vi "Main (429).vi"() -> ()   [LabVIEW 2020]
doc: "Use this template to build a simple state machine design pattern. Each state executes code and determines which state to transition to."
uses:
  Controls/State.ctl
  Controls/Data.ctl
  Controls/Database_Array.ctl
  Controls/Encoding.ctl
  <vilib>/Utility/error.llb/DialogType.ctl
  <userlib>/_OpenG.lib/array/array.llb/Remove Duplicates from 1D Array (I32)__ogtk.vi
  <userlib>/_OpenG.lib/array/array.llb/Sort 1D Array (I32)__ogtk.vi
  <userlib>/_OpenG.lib/array/array.llb/Search 1D Array (I32)__ogtk.vi
  <userlib>/_OpenG.lib/array/array.llb/Index 1D Array Elements (Variant)__ogtk.vi
  Libraries/Ballard_429_Parameter_ni/Ballard_429_Parameter_ni.lvlib
  Libraries/Aim_429_Parameter_ni/AIM_429_Parameter_ni.lvlib
panel:
  in  "formatting":enum16{"NIVeriStandAdd-Ons", "ni", "ni-AIM"}(ring)
  in  "Configure SelfTestBus?":bool
  out "Progress":string
  in  "Stop Button":bool
  in  "Generate XMLs":bool
  in  "Database Filepath (xlsx)":path
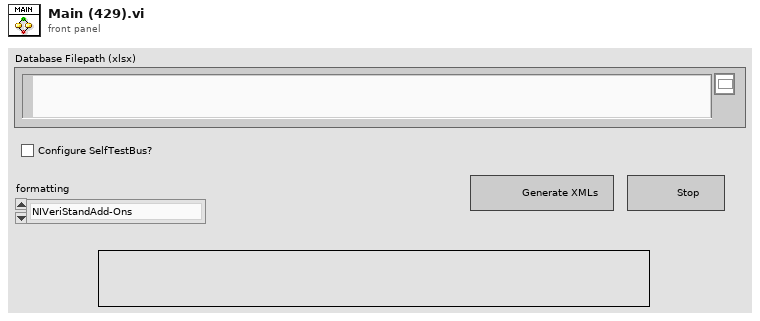
[diagram p1: front panel]
types:
  T1 = typedef "DialogType.ctl" = u16
  T2 = typedef "Data.ctl" = cluster{"Cores to Process Array":i32[], "All Parameters Array":T3[], "Filtered Parameter Array":T3[], "Core Number":i32, "Database Filepath (xlsx)":path, "Selected Self Test Channels":i32[], "formatting":enum16{"NIVeriStandAdd-Ons", "ni", "ni-AIM"}}
  T3 = typedef "Database_Array.ctl" = cluster{"Core Number":i32, "Channel Number":i32, "Channel Name":string, "Channel Speed":i32, "Label Decimal":i32, "Label Name":string, "Min Rate (mS)":i32, "Max Rate (mS)":i32, "SDI":i32, "SSM":i32, "Create SDI":bool, "Create SSM":bool, "Create Parity":bool, "Parameter Name":string, "Start Bit":i32, "Number of Bits":i32, "Scale":string, "Offset":string, "Signed":bool, "Unit":string, "Encoding":T4, "Default Value":string}
  T4 = typedef "Encoding.ctl" = enum16{"BCD", "BNR", "Discrete"}
  T5 = typedef "State.ctl" = enum16{"Initialize", "Wait for Event", "Read Database File", "Get Core Data", "Write HW XML File", "Write Parameter XML File", "Exit"}
  T6 = enum8{"Enabled", "Disabled", "Disabled and Grayed Out"}
  T7 = enum32{"invalid app kind", "Development System", "Run Time System", "Student Edition", "Embedded LabVIEW", "Evaluation", "Custom"}
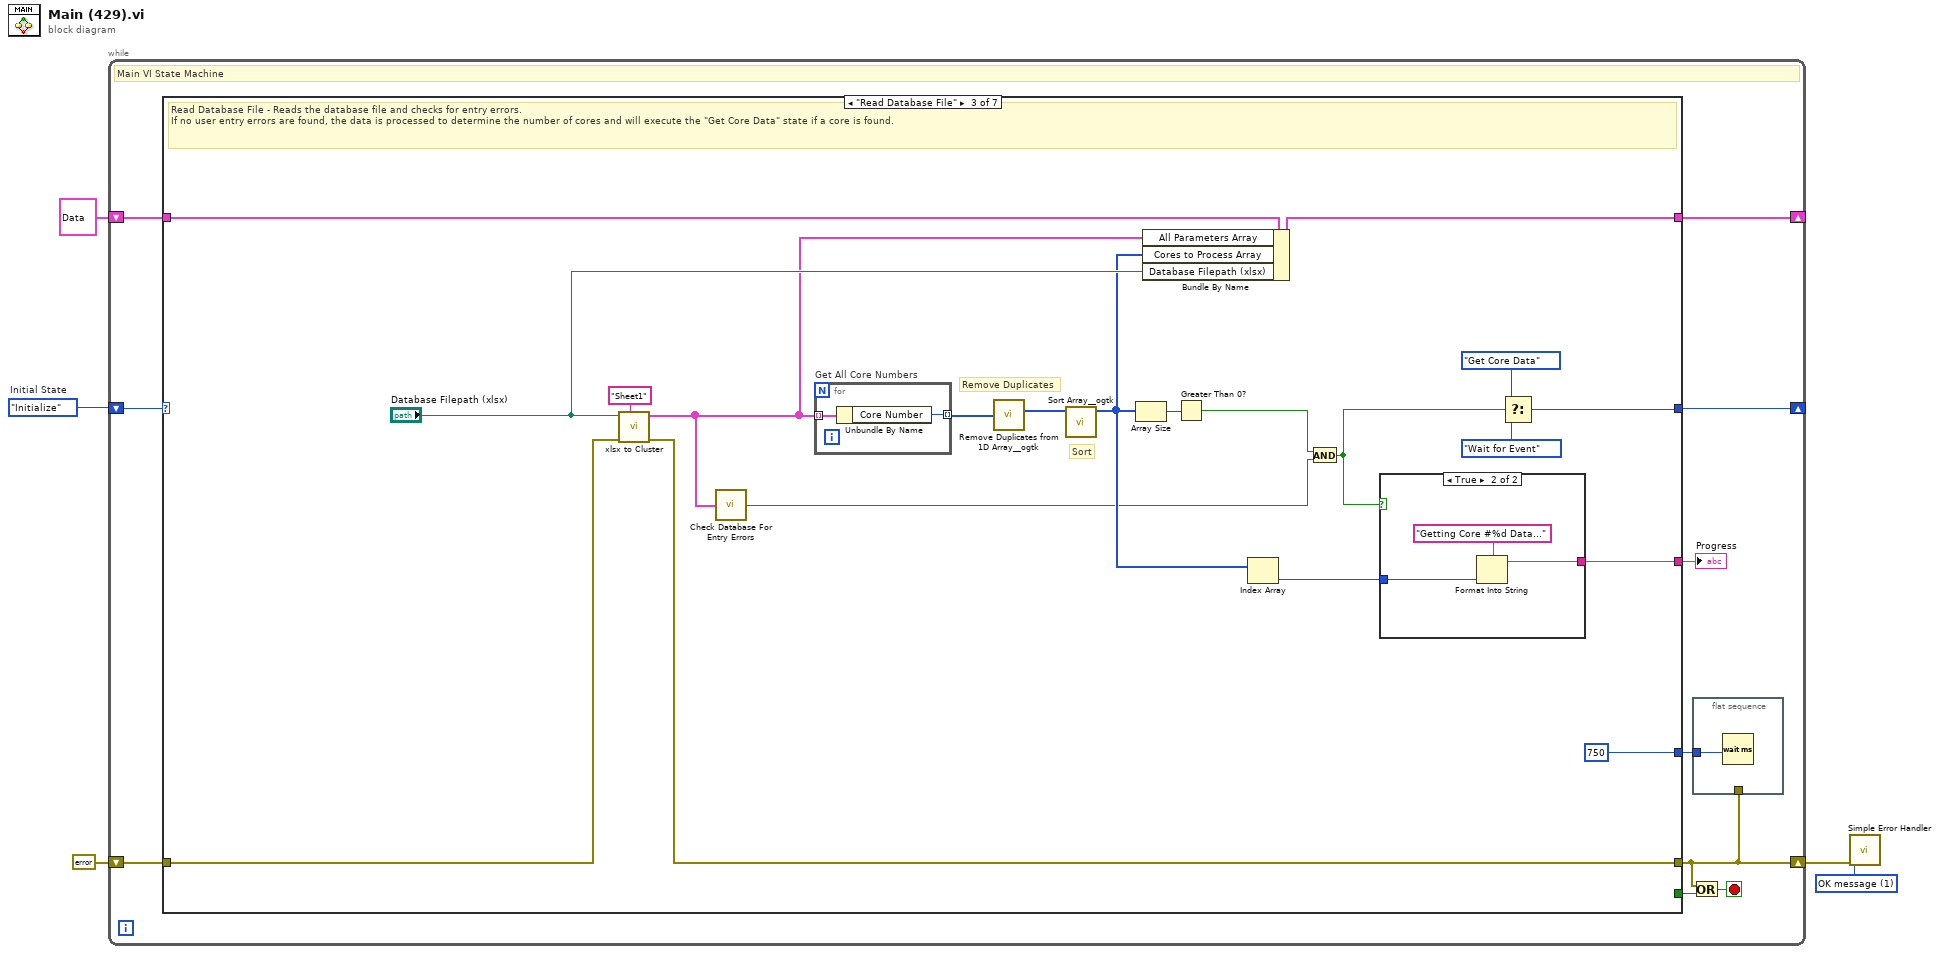
[diagram p0: block diagram]
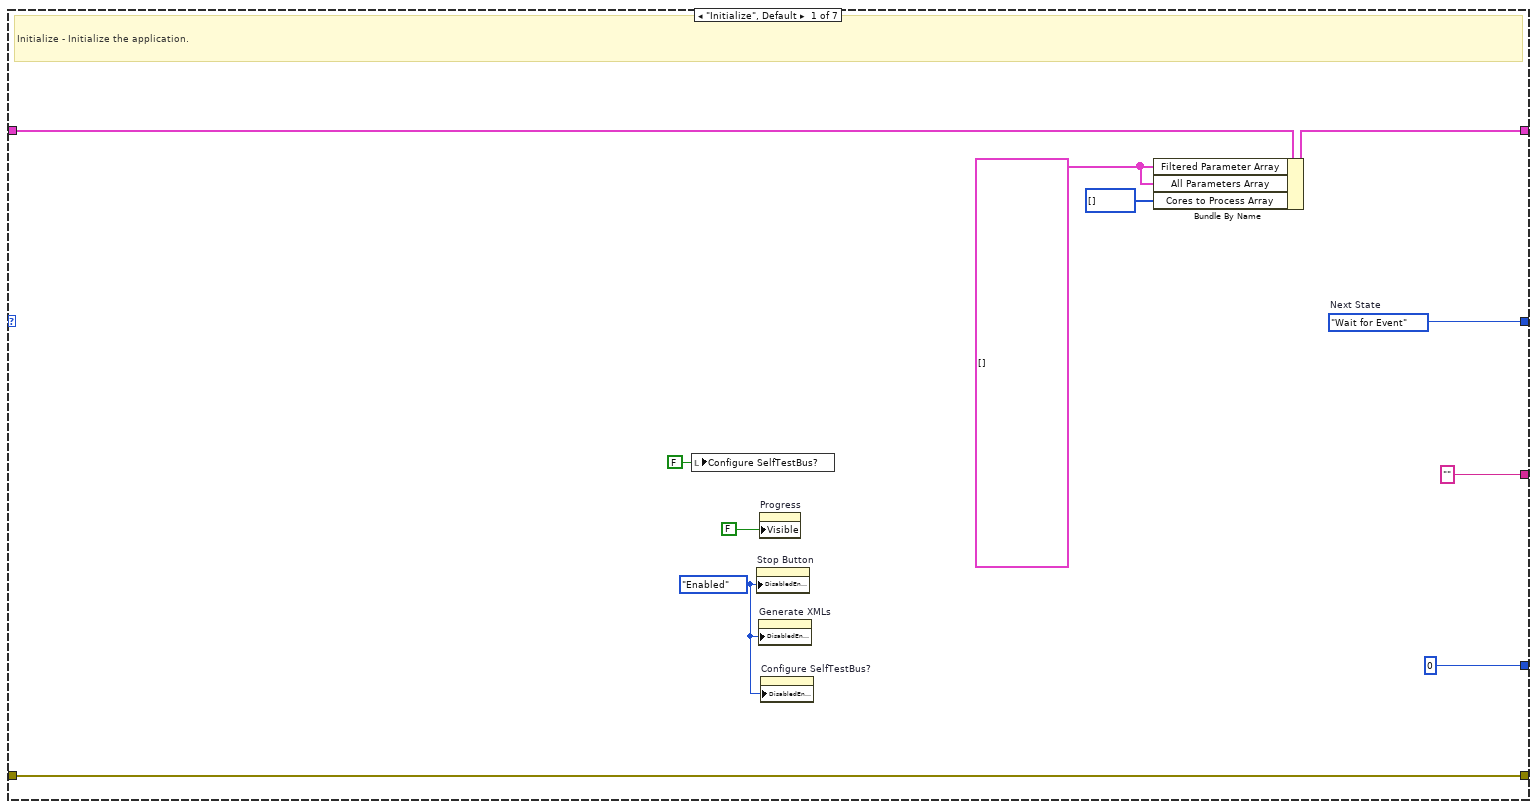
[diagram p2: hidden frame]
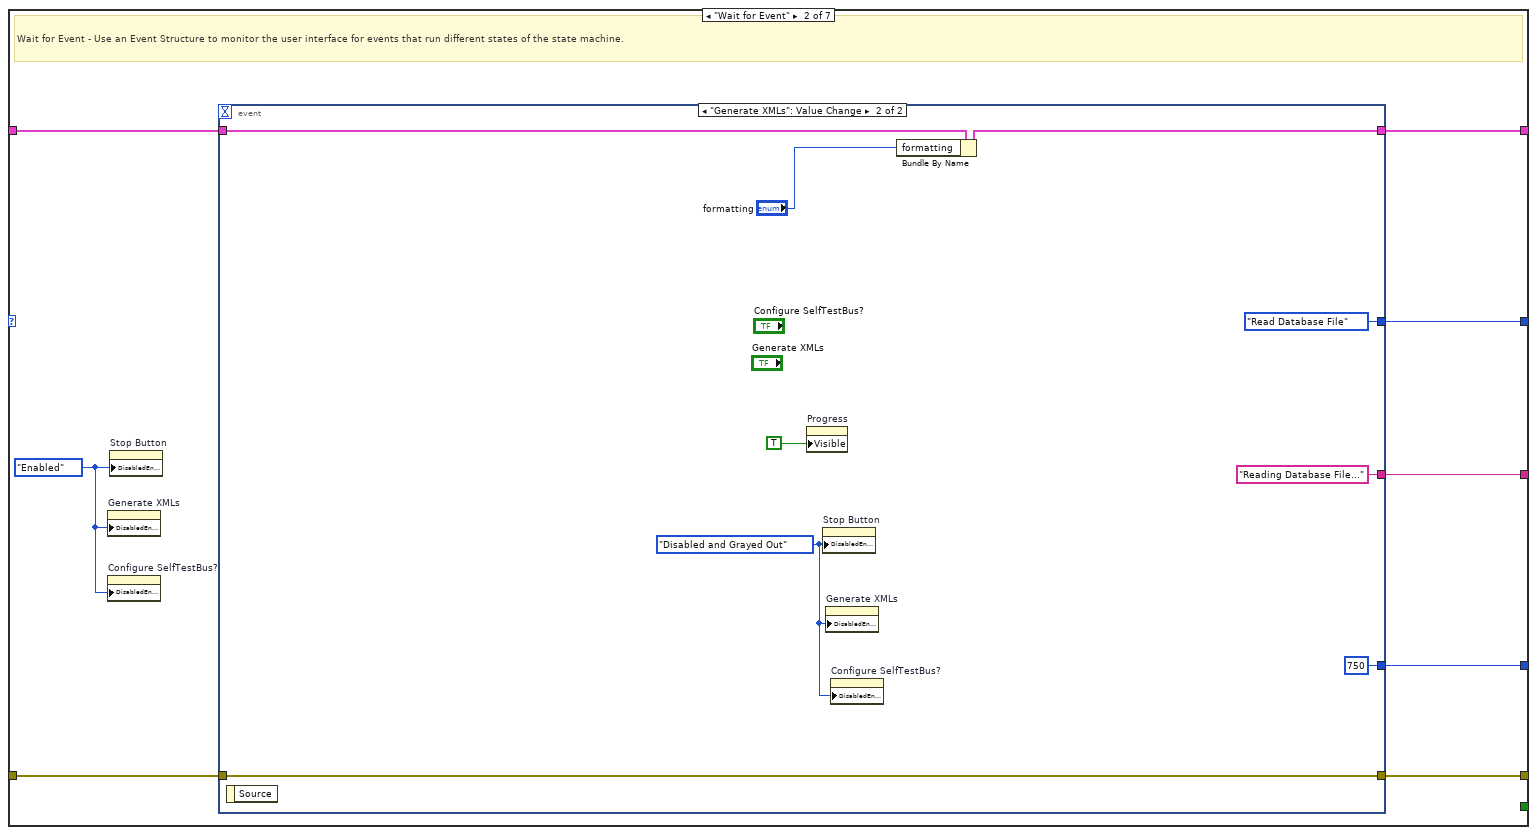
[diagram p3: hidden frame]
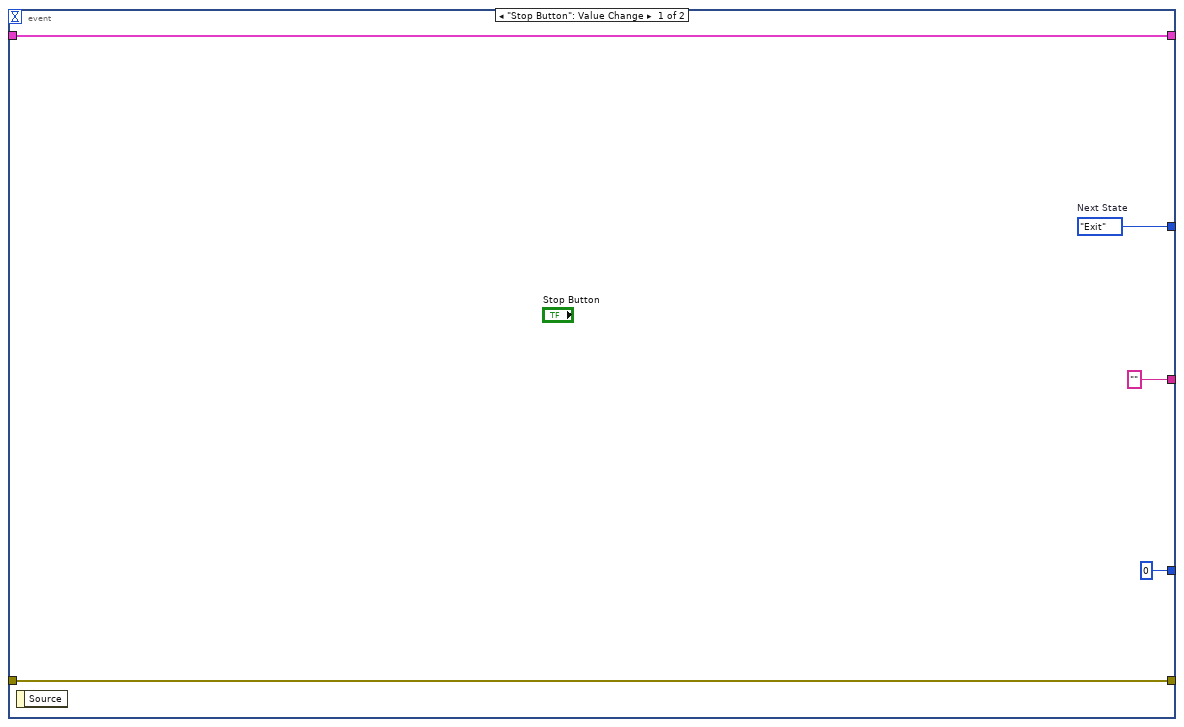
[diagram p4: hidden frame]
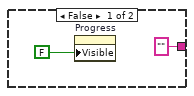
[diagram p5: hidden frame]
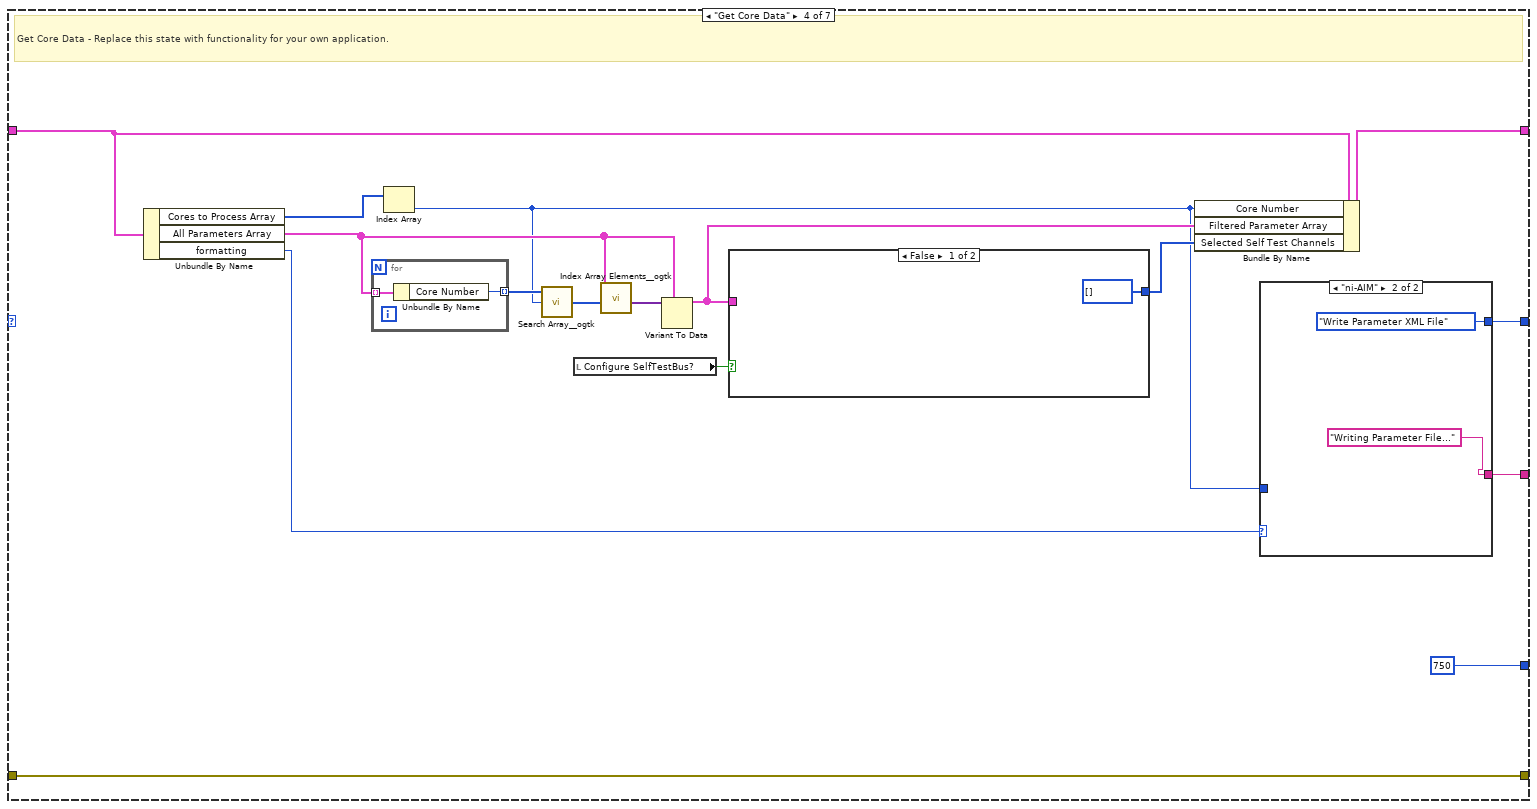
[diagram p6: hidden frame]
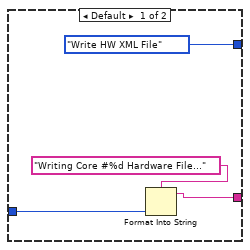
[diagram p7: hidden frame]
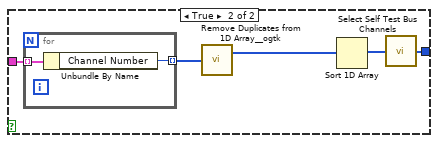
[diagram p8: hidden frame]
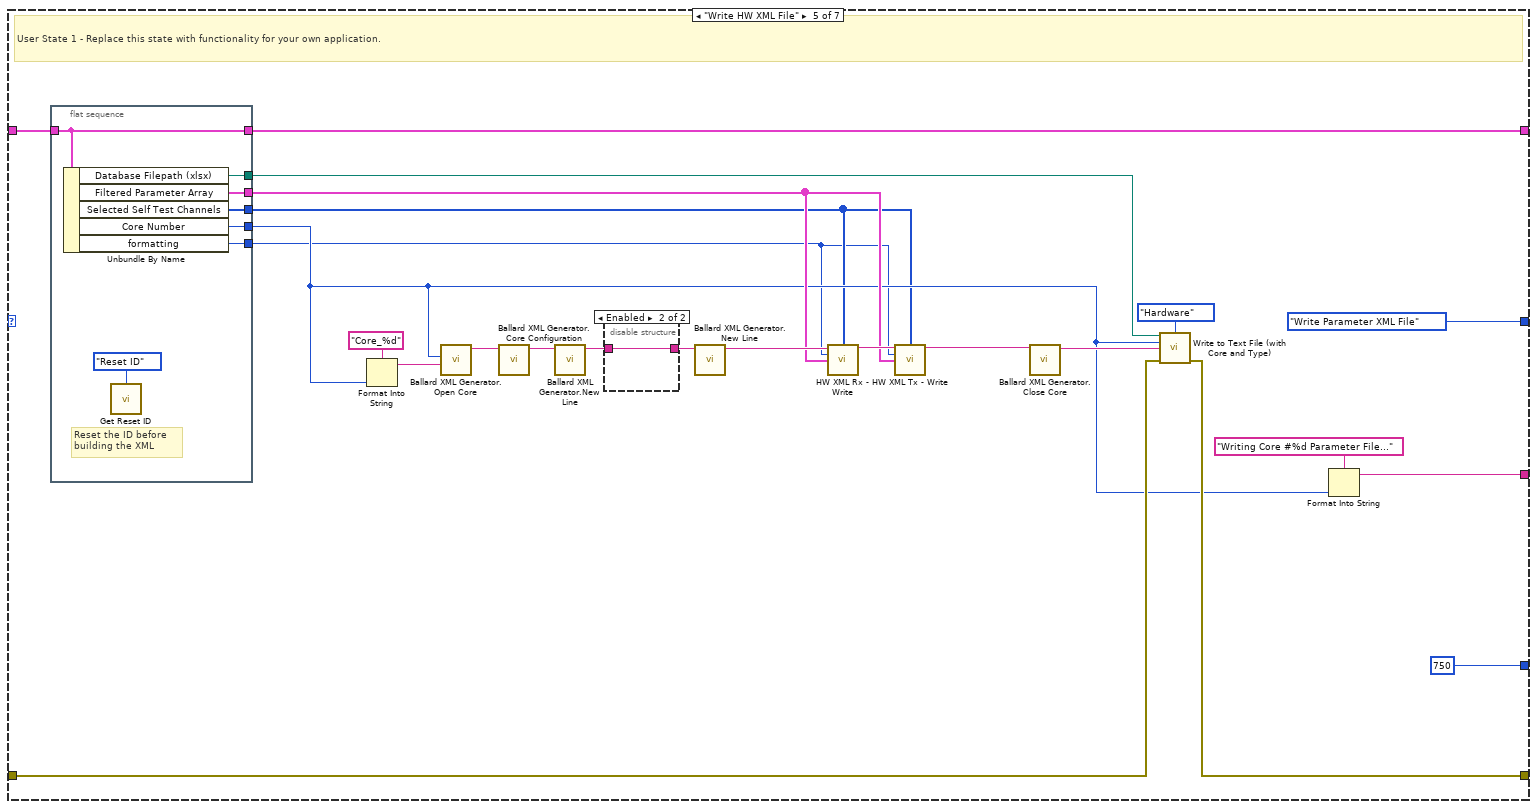
[diagram p9: hidden frame]
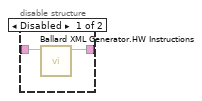
[diagram p10: hidden frame]
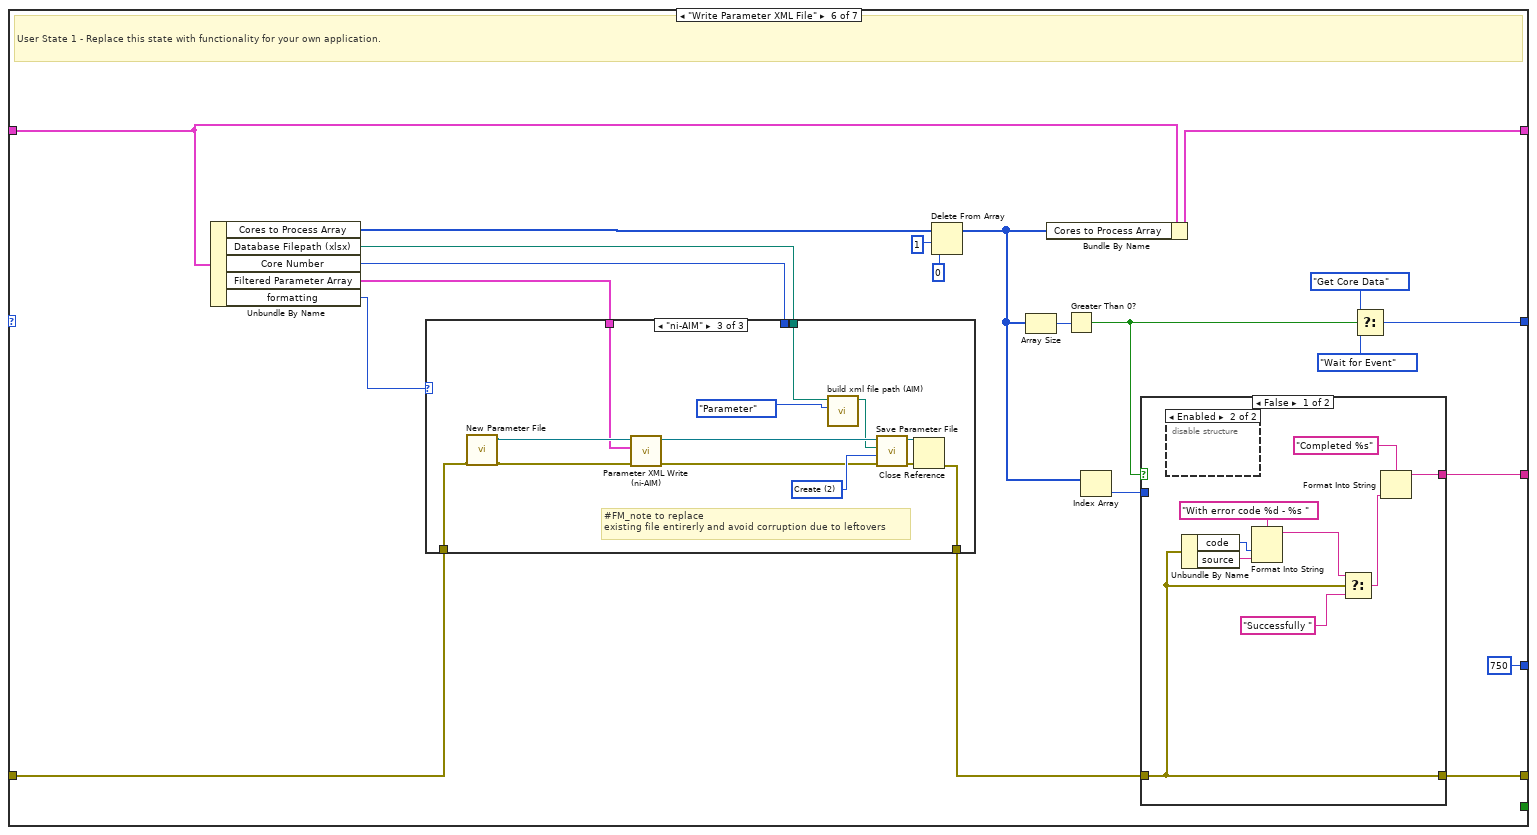
[diagram p11: hidden frame]
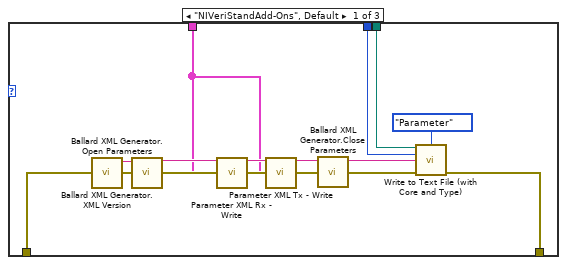
[diagram p12: hidden frame]
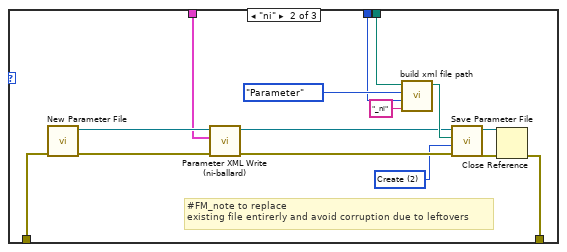
[diagram p13: hidden frame]
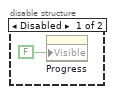
[diagram p14: hidden frame]
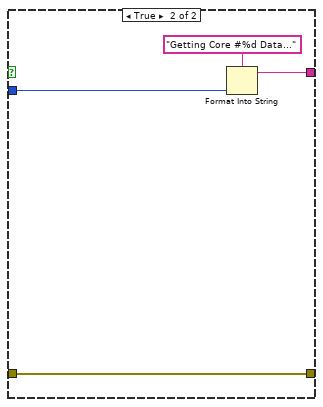
[diagram p15: hidden frame]
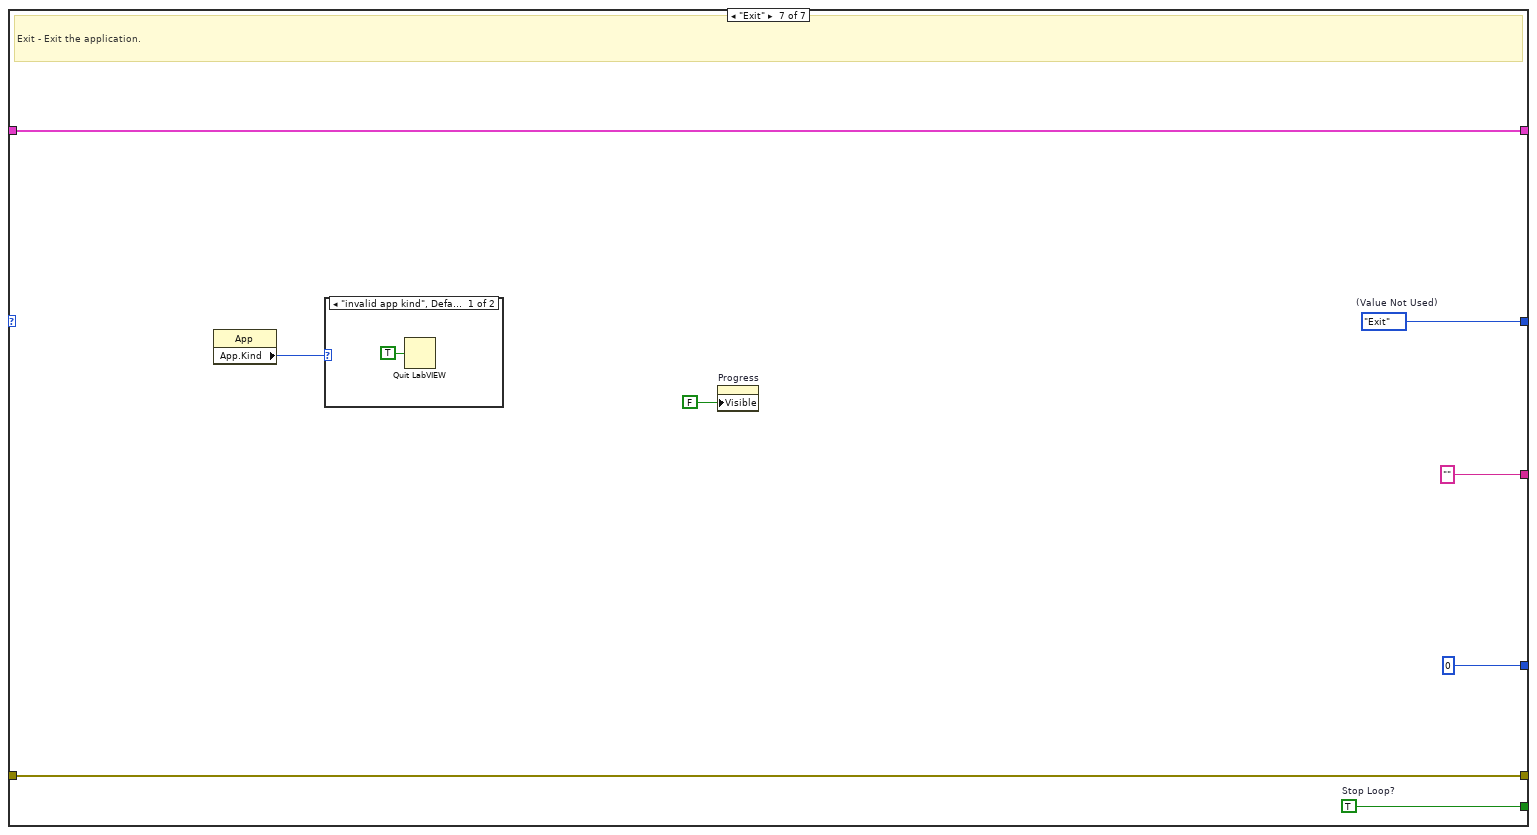
[diagram p16: hidden frame]
diagram:
  w1 = T1 1 items=["no dialog", "OK message", "continue or stop message", "OK message + warnings", "continue/stop + warnings"] ("type of dialog (OK msg:1)")
  w5 = State."Initialize"  # Initial State
  n1 = while {
    shift-right: [w14] -> _
    shift-left: w5 -> [w15]
    shift-right: [w12] -> _
    shift-left: T2 {"Cores to Process Array"=[], "All Parameters Array"=[], "Filtered Parameter Array"=[], "Core Number"=0, "Database Filepath (xlsx)"=path "C:/Users/jkreienh/Desktop/Preliminary Ballard Database Template.xlsx", "Selected Self Test Channels"=[], "formatting"=enum."NIVeriStandAdd-Ons"} ("Data") -> [w13]
    shift-right: [w7] -> w2
    shift-left: errorcluster {"status"=FALSE, "code"=0, "source"=""} ("error constant") -> [w11]
    stop <- w9 stop-if-true
    # "Main VI State Machine"
    n2 = case shown="\"Read Database File\"" w15 {
      tunnel: [w27 w35 w60 w86 State."Write Parameter XML File" ("Next State") w159 w224] -> w14
      tunnel: [_ _ _ _ _ _ w222] -> w10
      tunnel: w13 -> [w25 w34 w65 w90 w117 w156 w223]
      tunnel: [w24 w33 w64 w83 w116 w155 w223] -> w12
      tunnel: w11 -> [w26 w32 w57 w85 w120 w163 w221]
      tunnel: [w26 w31 w68 w85 w119 w144 w221] -> w7
      tunnel: ["" w30 w56 w77 w113 w151 ""] -> w8
      tunnel: [u32 0 ("milliseconds to wait") w29 u32 750 ("milliseconds to wait") u32 750 ("milliseconds to wait") u32 750 ("milliseconds to wait") u32 750 ("milliseconds to wait") u32 0 ("milliseconds to wait")] -> w6
      frame "Initialize", Default {
        w18 = T6."Enabled" ("Disabled")
        w22 = T3[] [] ("Parameter Array")
        w27 = State."Wait for Event"  # Next State
        # "Initialize - Initialize the application."
        n3 = local write "Configure SelfTestBus?"(FALSE ("Configure SelfTestBus?")) -> ()
        n4 = property on="Stop Button" class="Bool"("DisabledEnum"=w18) -> ()  [unwired: 2 in, 2 out]
        n5 = property on="Generate XMLs" class="Bool"("DisabledEnum"=w18) -> ()  [unwired: 2 in, 2 out]
        n6 = property on="Progress" class="Str"("Visible"=FALSE) -> ()  [unwired: 2 in, 2 out]
        n7 = property on="Configure SelfTestBus?" class="Bool (strict)"("DisabledEnum"=w18) -> ()  [unwired: 2 in, 2 out]
        n8 = Bundle By Name(cluster=w25, "Filtered Parameter Array"=w22, "All Parameters Array"=w22, "Cores to Process Array"=i32[] [] ("Core Array")) -> (w24:T2)
      }
      frame "Wait for Event" {
        w28 = T6."Enabled" ("Disabled")
        # "Wait for Event - Use an Event Structure to monitor the user interface for events that run different states of the state machine."
        n9 = property on="Generate XMLs" class="Bool"("DisabledEnum"=w28) -> ()  [unwired: 2 in, 2 out]
        n10 = property on="Configure SelfTestBus?" class="Bool (strict)"("DisabledEnum"=w28) -> ()  [unwired: 2 in, 2 out]
        n11 = property on="Stop Button" class="Bool"("DisabledEnum"=w28) -> ()  [unwired: 2 in, 2 out]
        n12 = event shown="[1] \"Generate XMLs\": Value Change" {
          selector: _ -> [_ _]
          dyn-events: _ -> [_ _]
          timeout: _ -> [_ _]
          tunnel: [w40 State."Read Database File" ("Next State")] -> w35
          tunnel: w34 -> [w39 w49]
          tunnel: [w39 w42] -> w33
          tunnel: w32 -> [w38 w48]
          tunnel: [w38 w48] -> w31
          tunnel: ["" "Reading Database File..."] -> w30
          tunnel: [u32 0 ("milliseconds to wait") u32 750 ("milliseconds to wait")] -> w29
          event "Stop Button": Value Change {
            w40 = State."Exit"  # Next State
            n13 = event-data() -> ()  [unwired: 1 in, 1 out]
          }
          event "Generate XMLs": Value Change {
            w43 = T6."Disabled and Grayed Out" ("Disabled")
            n14 = event-data() -> ()  [unwired: 1 in, 1 out]
            n15 = property on="Progress" class="Str"("Visible"=TRUE) -> ()  [unwired: 2 in, 2 out]
            n16 = property on="Stop Button" class="Bool"("DisabledEnum"=w43) -> ()  [unwired: 2 in, 2 out]
            n17 = property on="Generate XMLs" class="Bool"("DisabledEnum"=w43) -> ()  [unwired: 2 in, 2 out]
            n18 = property on="Configure SelfTestBus?" class="Bool (strict)"("DisabledEnum"=w43) -> ()  [unwired: 2 in, 2 out]
            n19 = Bundle By Name(cluster=w49, "formatting"="formatting") -> (w42:T2)
          }
        }
      }
      frame "Read Database File" {
        # "Sort"
        # "Remove Duplicates"
        # "Read Database File - Reads the database file and checks for entry errors. \nIf no user entry errors are found, the data is processed to determine the number of cores and will execute the \"Get Core Data\" state if a core is found."
        n20 = call "xlsx to Cluster.vi"("Excel._SheetName"="Sheet1", "Error (in)"=w57, "file path (dialog if empty)"="Database Filepath (xlsx)") -> ("Error (out)"=w68:errorcluster, "Parameter Array"=w58:T3[])  [unwired: 7 in]
        n21 = call "Check Database For Entry Errors.vi"("All Parameters Array"=w58) -> ("Database OK?"=w51:bool)  [unwired: 14 in]
        n22 = for "Get All Core Numbers" {
          tunnel: w58 -> [w76] mode=indexing
          tunnel: [w75] -> w67 mode=indexing
          n23 = Unbundle By Name(w76) -> ("Core Number"=w75:i32)
        }
        n24 = call-poly <userlib>:"Remove Duplicates from 1D Array__ogtk.vi"("Input Array"=w67) -> ("Output Array"=w66:i32[])  [unwired: 1 out]
        n25 = call-poly <userlib>:"Sort Array__ogtk.vi"("Array in"=w66) -> ("Sorted Array out"=w55:i32[])  [unwired: 9 in, 1 out]
        n26 = Array Size(array=w55) -> (size(s)=w63:i32)
        n27 = Bundle By Name(cluster=w65, "All Parameters Array"=w58, "Cores to Process Array"=w55, "Database Filepath (xlsx)"="Database Filepath (xlsx)") -> (w64:T2)
        n28 = Greater Than 0?(x=w63) -> (x > 0?=w52:bool)
        n29 = Index Array(array=w55) -> (element=w54:i32)  [unwired: 1 in]
        n30 = And(x=w52, y=w51) -> (x .and. y?=w50:bool)
        n31 = case shown="True" w50 {
          tunnel: ["" ("f") w73] -> w56
          tunnel: w54 -> [_ w74]
          frame False {
            n32 = property on="Progress" class="Str"("Visible"=FALSE) -> ()  [unwired: 2 in, 2 out]
          }
          frame True {
            n33 = Format Into String(format string="Getting Core #%d Data..." ("String"), w74) -> (resulting string=w73:string)  [unwired: 2 in, 1 out]
          }
        }
        n34 = Select(t=State."Get Core Data", s=w50, f=State."Wait for Event") -> (s? t:f=w60:T5)
      }
      frame "Get Core Data" {
        # "Get Core Data - Replace this state with functionality for your own application."
        n35 = Unbundle By Name(w90) -> ("Cores to Process Array"=w87:i32[], "All Parameters Array"=w89:T3[], "formatting"=w79:enum16{"NIVeriStandAdd-Ons", "ni", "ni-AIM"})
        n36 = for {
          tunnel: w89 -> [w108] mode=indexing
          tunnel: [w107] -> w92 mode=indexing
          n37 = Unbundle By Name(w108) -> ("Core Number"=w107:i32)
        }
        n38 = Index Array(array=w87) -> (element=w78:i32)  [unwired: 1 in]
        n39 = call-poly <userlib>:"Search Array__ogtk.vi"("Array"=w92, "Element Data"=w78) -> ("Indices of Elements"=w91:i32[])  [unwired: 7 in]
        n40 = local read "Configure SelfTestBus?"() -> (w80:bool)
        n41 = call-poly <userlib>:"Index Array Elements__ogtk.vi"("indices"=w91, "array"=w89) -> ("elements"=w88:variant[])  [unwired: 9 in]
        n42 = Variant To Data(type=w89, Variant=w88) -> (data=w82:T3[])  [unwired: 1 in, 1 out]
        n43 = case shown="False" w80 {
          tunnel: w82 -> [_ w103]
          tunnel: [i32[] [] ("Selected Channels") w100] -> w81
          frame False {
          }
          frame True {
            n44 = for {
              tunnel: [w106] -> w102 mode=indexing
              tunnel: w103 -> [w105] mode=indexing
              n45 = Unbundle By Name(w105) -> ("Channel Number"=w106:i32)
            }
            n46 = call-poly <userlib>:"Remove Duplicates from 1D Array__ogtk.vi"("Input Array"=w102) -> ("Output Array"=w104:i32[])  [unwired: 1 out]
            n47 = Sort 1D Array(array=w104) -> (sorted array=w101:i32[])
            n48 = call "Select Self Test Bus Channels.vi"("Channels"=w101) -> ("Selected Channels"=w100:i32[])  [unwired: 14 in]
          }
        }
        n49 = Bundle By Name(cluster=w90, "Core Number"=w78, "Filtered Parameter Array"=w82, "Selected Self Test Channels"=w81) -> (w83:T2)
        n50 = case shown="\"ni-AIM\"" w79 {
          tunnel: [State."Write HW XML File" State."Write Parameter XML File"] -> w86
          tunnel: w78 -> [w94 _]
          tunnel: [w93 "Writing Parameter File..." ("String")] -> w77
          frame Default {
            n51 = Format Into String(format string="Writing Core #%d Hardware File..." ("String"), w94) -> (resulting string=w93:string)  [unwired: 2 in, 1 out]
          }
          frame "ni-AIM" {
          }
        }
      }
      frame "Write HW XML File" {
        # "User State 1 - Replace this state with functionality for your own application."
        n52 = flat-sequence {
          tunnel: [w139] -> w122
          tunnel: w117 -> [w137]
          tunnel: [w137] -> w116
          tunnel: [w136] -> w115
          tunnel: [w135] -> w111
          tunnel: [w134] -> w110
          tunnel: [w133] -> w109
          frame #0 {
            # "Reset the ID before building the XML"
            n53 = Unbundle By Name(w137) -> ("Database Filepath (xlsx)"=w136:path, "Filtered Parameter Array"=w139:T3[], "Selected Self Test Channels"=w134:i32[], "Core Number"=w135:i32, "formatting"=w133:enum16{"NIVeriStandAdd-Ons", "ni", "ni-AIM"})
            n54 = call "Get Reset ID.vi"("Function"=enum16{"Get ID", "Reset ID"}."Reset ID") -> ()  [unwired: 14 in, 1 out]
          }
        }
        n55 = Format Into String(format string="Core_%d", w111) -> (resulting string=w123:string)  [unwired: 2 in, 1 out]
        n56 = call "Ballard XML Generator.Open Core.vi"("name"=w123, "id"=w111) -> ("string out"=w125:string)  [unwired: 9 in]
        n57 = call "Ballard XML Generator.Core Configuration.vi"("string in"=w125) -> ("string out"=w126:string)  [unwired: 10 in]
        n58 = call "Ballard XML Generator.New Line.vi"("string in"=w126) -> ("string out"=w127:string)  [unwired: 10 in]
        n59 = disable-structure shown="Enabled" {
          disable-tunnel: w127 -> [w141 w142]
          disable-tunnel: [w140 w142] -> w128
          frame Disabled {
            n60 = call "Ballard XML Generator.HW Instructions.vi"("string in"=w141) -> ("string out"=w140:string)  [unwired: 10 in]
          }
          frame Enabled {
          }
        }
        n61 = call "Ballard XML Generator.New Line.vi"("string in"=w128) -> ("string out"=w129:string)  [unwired: 10 in]
        n62 = call "HW XML Rx - Write.vi"("String (in)"=w129, "Selected Channels"=w110, "formatting (NIVeriStandAdd-Ons)"=w109, "Parameter Array"=w122) -> ("String (out)"=w130:string)  [unwired: 11 in]
        n63 = call "HW XML Tx - Write.vi"("String (in)"=w130, "Selected Channels"=w110, "formatting (NIVeriStandAdd-Ons)"=w109, "Parameter Array"=w122) -> ("String (out)"=w131:string)  [unwired: 11 in]
        n64 = call "Ballard XML Generator.Close Core.vi"("string in"=w131) -> ("string out"=w118:string)  [unwired: 10 in]
        n65 = call "Write to Text File (with Core and Type).vi"("Database Filepath (xlsx)"=w115, "Filetype"=enum16{"Hardware", "Parameter"}."Hardware", "Core"=w111, "Text"=w118, "Error (in)"=w120) -> ("Error (out)"=w119:errorcluster)  [unwired: 10 in]
        n66 = Format Into String(format string="Writing Core #%d Parameter File..." ("String"), w111) -> (resulting string=w113:string)  [unwired: 2 in, 1 out]
      }
      frame "Write Parameter XML File" {
        # "User State 1 - Replace this state with functionality for your own application."
        n67 = Unbundle By Name(w156) -> ("Cores to Process Array"=w157:i32[], "Database Filepath (xlsx)"=w153:path, "Core Number"=w150:i32, "Filtered Parameter Array"=w154:T3[], "formatting"=w143:enum16{"NIVeriStandAdd-Ons", "ni", "ni-AIM"})
        n68 = case shown="\"ni-AIM\"" w143 {
          tunnel: w163 -> [w170 w189 w201]
          tunnel: [w169 w188 w202] -> w145
          tunnel: w154 -> [w166 w179 w196]
          tunnel: w153 -> [w165 w184 w192]
          tunnel: w150 -> [w164 w183 _]
          frame "NIVeriStandAdd-Ons", Default {
            n69 = call "Ballard XML Generator.XML Version.vi"() -> ("string out"=w174:string)  [unwired: 11 in]
            n70 = call "Ballard XML Generator.Open Parameters.vi"("string in"=w174) -> ("string out"=w173:string)  [unwired: 10 in]
            n71 = call "Parameter XML Rx - Write.vi"("String (in)"=w173, "Parameter Array"=w166) -> ("String (out)"=w172:string)  [unwired: 13 in]
            n72 = call "Parameter XML Tx - Write.vi"("String (in)"=w172, "Parameter Array"=w166) -> ("String (out)"=w171:string)  [unwired: 13 in]
            n73 = call "Ballard XML Generator.Close Parameters.vi"("string in"=w171) -> ("string out"=w168:string)  [unwired: 10 in]
            n74 = call "Write to Text File (with Core and Type).vi"("Database Filepath (xlsx)"=w165, "Filetype"=enum16{"Hardware", "Parameter"}."Parameter", "Core"=w164, "Text"=w168, "Error (in)"=w170) -> ("Error (out)"=w169:errorcluster)  [unwired: 10 in]
          }
          frame "ni" {
            w175 = 2 items=["CreateNew"=1, "Create"=2, "Open"=3, "OpenOrCreate"=4, "Truncate"=5, "Append"=6] ("mode (Create)")
            # "#FM_note to replace \nexisting file entirerly and avoid corruption due to leftovers"
            n75 = call "New Parameter File.vi"("error in"=w189) -> ("error out"=w180:errorcluster, "new parameter file"=w181:refnum<k24>)  [unwired: 9 in]
            n76 = call "Parameter XML Write (ni-ballard).vi"("error in"=w180, "Parameter Array"=w179, "parameter file in"=w181) -> ("error out"=w177:errorcluster, "parameter file out"=w178:refnum<k24>)  [unwired: 7 in]
            n77 = call "build xml file path.vi"("additional string(\"\")"="_ni" ("additional string(\"\")"), "Core"=w183, "Filetype"=enum16{"Hardware", "Parameter"}."Parameter", "Database Filepath in"=w184) -> ("xml path out"=w182:path)  [unwired: 7 in]
            n78 = call "Save Parameter File.vi"("error in"=w177, "mode (Create)"=w175, "XML path"=w182, "parameter file in"=w178) -> ("error out"=w187:errorcluster, "parameter file out"=w186:refnum<k24>)  [unwired: 5 in, 1 out]
            n79 = Close Reference(reference=w186, error in (no error)=w187) -> (error out=w188:errorcluster)
          }
          frame "ni-AIM" {
            w199 = 2 items=["CreateNew"=1, "Create"=2, "Open"=3, "OpenOrCreate"=4, "Truncate"=5, "Append"=6] ("mode (Create)")
            # "#FM_note to replace \nexisting file entirerly and avoid corruption due to leftovers"
            n80 = call "New Parameter File.vi"("error in"=w201) -> ("error out"=w193:errorcluster, "new parameter file"=w197:refnum<k24>)  [unwired: 9 in]
            n81 = call "Parameter XML Write (ni-AIM).vi"("error in"=w193, "Parameter Array"=w196, "parameter file in"=w197) -> ("error out"=w194:errorcluster, "parameter file out"=w195:refnum<k24>)  [unwired: 7 in]
            n82 = call "build xml file path (AIM).vi"("Filetype"=enum16{"Hardware", "Parameter"}."Parameter", "Database Filepath in"=w192) -> ("xml path out"=w190:path)  [unwired: 9 in]
            n83 = call "Save Parameter File.vi"("error in"=w194, "mode (Create)"=w199, "XML path"=w190, "parameter file in"=w195) -> ("error out"=w198:errorcluster, "parameter file out"=w200:refnum<k24>)  [unwired: 5 in, 1 out]
            n84 = Close Reference(reference=w200, error in (no error)=w198) -> (error out=w202:errorcluster)
          }
        }
        n85 = Delete From Array(array=w157, length=1, index=0) -> (array with subset deleted=w148:i32[])  [unwired: 1 out]
        n86 = Array Size(array=w148) -> (size(s)=w162:i32)
        n87 = Bundle By Name(cluster=w156, "Cores to Process Array"=w148) -> (w155:T2)
        n88 = Greater Than 0?(x=w162) -> (x > 0?=w149:bool)
        n89 = Index Array(array=w148) -> (element=w147:i32)  [unwired: 1 in]
        n90 = case shown="False" w149 {
          tunnel: [w210 w215] -> w151
          tunnel: w147 -> [_ w214]
          tunnel: w145 -> [w203 w213]
          tunnel: [w203 w213] -> w144
          frame False {
            n91 = disable-structure shown="Enabled" {
              frame Disabled {
                n92 = property on="Progress" class="Str"("Visible"=FALSE) -> ()  [unwired: 2 in, 2 out]
              }
              frame Enabled {
              }
            }
            n93 = Unbundle By Name(w203) -> ("code"=w208:i32, "source"=w207:string)
            n94 = Format Into String(format string="With error code %d - %s ", w208, w207) -> (resulting string=w205:string)  [unwired: 2 in, 1 out]
            n95 = Select(t=w205, s=w203, f="Successfully ") -> (s? t:f=w206:string)
            n96 = Format Into String(format string="Completed %s", w206) -> (resulting string=w210:string)  [unwired: 2 in, 1 out]
          }
          frame True {
            n97 = Format Into String(format string="Getting Core #%d Data..." ("String"), w214) -> (resulting string=w215:string)  [unwired: 2 in, 1 out]
          }
        }
        n98 = Select(t=State."Get Core Data" ("Next State"), s=w149, f=State."Wait for Event" ("Next State")) -> (s? t:f=w159:T5)
      }
      frame "Exit" {
        w222 = TRUE  # Stop Loop?
        w224 = State."Exit"  # (Value Not Used)
        # "Exit - Exit the application."
        n99 = property class="App"() -> ("App.Kind"=w217:T7)  [unwired: 2 in, 2 out]
        n100 = case shown="\"invalid app kind\", Default" w217 {
          frame "invalid app kind", Default {
            n101 = Quit LabVIEW(quit? (T)=TRUE) -> ()
          }
          frame "Development System" {
          }
        }
        n102 = property on="Progress" class="Str"("Visible"=FALSE) -> ()  [unwired: 2 in, 2 out]
      }
    }
    "Progress" <- w8
    n103 = Or(x=w7, y=w10) -> (x .or. y?=w9:bool)
    n104 = flat-sequence {
      tunnel: w7 -> [_]
      tunnel: w6 -> [w16]
      frame #0 {
        n105 = Wait (ms)(milliseconds to wait=w16) -> ()  [unwired: 1 out]
      }
    }
  }
  n106 = call <vilib>:"Simple Error Handler.vi"("type of dialog (OK msg:1)"=w1, "error in (no error)"=w2) -> ()  [unwired: 3 in, 5 out]
